vi "CS POLARIS BME DG.configure objects.vi"(8 "error in (no error)":errorcluster, 11 "BME_DG_System in":refnum<class "BME_DG_System.lvclass">) -> (0 "error out":errorcluster, 3 "BME_DG_System out":refnum<class "BME_DG_System.lvclass">)   [LabVIEW 2009, in "CS POLARIS BME DG.lvlib"]
uses:
  CS POLARIS BME DG.lvlib
  LV-BME Interface/ChnlSettings.ctl
  DG Classes/BME_DG_G05P2/SG05P2 Clock and Trigger Settings.ctl
  LV-BME Interface/BME_DG_TriggerSettings.ctl
  LV-BME Interface/ClockSource.ctl
  DG Classes/BME_DG_System/BME_DG_System.lvclass
  ChnlParam.ctl
  DG Classes/BME_DG_Base/BME_DG_Base.lvclass
  DG Classes/BME_DG_Chnl/BME_DG_Chnl.lvclass
  POLARIS BME DG.lvlib
panel:
  in  "Karten Parameter":T1[](array[typedef])=[{"Trigger"={"InputTerminated?"=FALSE, "InternalClockPeriode(µs)"=1000000.0, "TriggerLevel"=1.25, "PresetValue"=0, "DivideBy"=1, "Clock Source"=1, "Gate Divider"=1, "PositiveGate?"=TRUE, "InternalTrigger?"=TRUE, "InternalArm?"=FALSE, "SWTrigger?"=FALSE, "RisingEdge?"=FALSE, "StopOnPreset?"=FALSE, "ResetWhenDone?"=TRUE, "TriggerEnabled?"=TRUE}, "ClockSource "=1, "V2 Trigger Settings"={"Gate Type"=TRUE, "Synchronize Gate"=FALSE, "Force Trigger (µs)"=0.0, "MS Bus"=16}, " prescaller crst oscill."=8, "CardName"="Master"}, {"Trigger"={"InputTerminated?"=TRUE, "InternalClockPeriode(µs)"=0.0, "TriggerLevel"=1.25, "PresetValue"=0, "DivideBy"=1, "Clock Source"=3, "Gate Divider"=1, "PositiveGate?"=TRUE, "InternalTrigger?"=FALSE, "InternalArm?"=FALSE, "SWTrigger?"=FALSE, "RisingEdge?"=FALSE, "StopOnPreset?"=FALSE, "ResetWhenDone?"=FALSE, "TriggerEnabled?"=FALSE}, "ClockSource "=4, "V2 Trigger Settings"={"Gate Type"=TRUE, "Synchronize Gate"=FALSE, "Force Trigger (µs)"=0.0, "MS Bus"=16}, " prescaller crst oscill."=1, "CardName"="S1"}, {"Trigger"={"InputTerminated?"=TRUE, "InternalClockPeriode(µs)"=0.0, "TriggerLevel"=1.25, "PresetValue"=0, "DivideBy"=1, "Clock Source"=3, "Gate Divider"=1, "PositiveGate?"=TRUE, "InternalTrigger?"=FALSE, "InternalArm?"=FALSE, "SWTrigger?"=FALSE, "RisingEdge?"=FALSE, "StopOnPreset?"=FALSE, "ResetWhenDone?"=FALSE, "TriggerEnabled?"=TRUE}, "ClockSource "=1, "V2 Trigger Settings"={"Gate Type"=TRUE, "Synchronize Gate"=FALSE, "Force Trigger (µs)"=0.0, "MS Bus"=16}, " prescaller crst oscill."=1, "CardName"="S2"}] {"V2 Trigger Settings"."MS Bus" format="%04x" items=["Local Primary"=1, "Local Secondary"=2, "Local Force"=4, "Resynchronize"=8, "Master Primary"=16, "Master Secondary"=32, "Master Force"=64, "System Clock"=128, "Delay Clock"=256, "Inhibit Local"=512, "Start Local"=1024, "Start Bus"=2048, "Step Back Local"=4096, "Step Back Bus"=8192, "Enable From E"=65536, "Enable From F"=131072, "Enable From Bus"=262144]; "V2 Trigger Settings"."Force Trigger (µs)" min=0.0 format="%.6f"; "ClockSource" items=["Internal Oscillator"=1, "External Trigger"=2, "Trigger & Oscillator"=3, "MasterSlave Bus"=4]; "Trigger"."Gate Divider" min=1 max=1000000; "Trigger"."Clock Source" items=["Internal Oscillator"=1, "External Trigger"=2, "Trigger & Oscillator"=3]; "Trigger"."InternalClockPeriode(µs)" format="%#_11g"}
  in  "ChnParam2write":T4={" Delay (µs)"=0.0, "On? (false)"=TRUE, "PositiveVoltage?"=TRUE, "50OhmTerminated? "=TRUE, "25OhmOutput?"=FALSE} {"Delay (µs)" min=0.0 max=100000000.0 format="%.5f"}
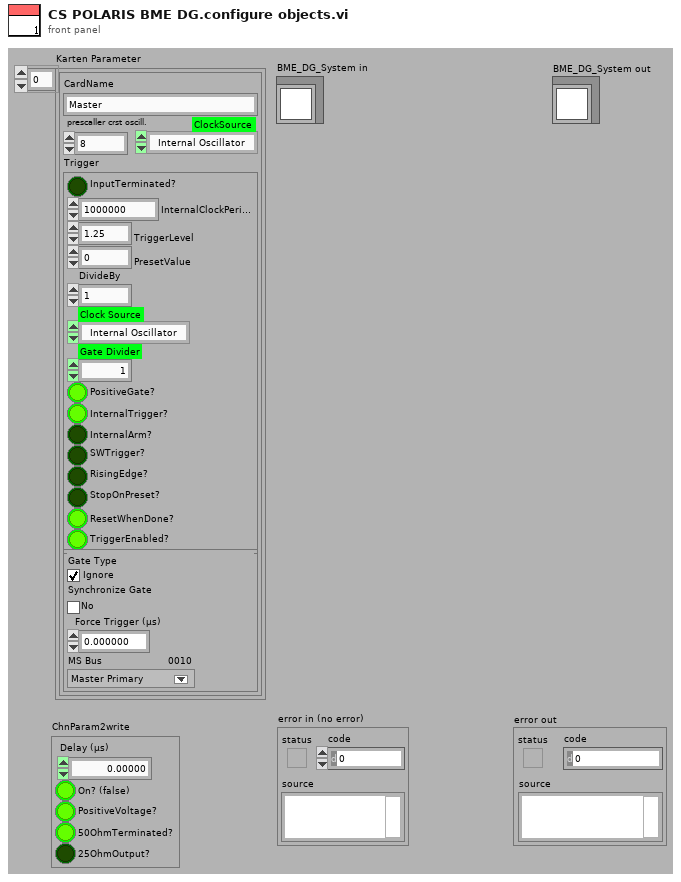
[diagram p1: front panel]
types:
  T1 = typedef "SG05P2 Clock and Trigger Settings.ctl" = cluster{"Trigger":T2, "ClockSource ":T3, "V2 Trigger Settings":cluster{"Gate Type":bool, "Synchronize Gate":bool, "Force Trigger (µs)":dbl, "MS Bus":u32}, " prescaller crst oscill.":u32, "CardName":string}
  T2 = typedef "POLARIS BME DG.lvlib/BME_DG_TriggerSettings.ctl" = cluster{"InputTerminated?":bool, "InternalClockPeriode(µs)":dbl, "TriggerLevel":dbl, "PresetValue":i32, "DivideBy":i32, "Clock Source":u32, "Gate Divider":i32, "PositiveGate?":bool, "InternalTrigger?":bool, "InternalArm?":bool, "SWTrigger?":bool, "RisingEdge?":bool, "StopOnPreset?":bool, "ResetWhenDone?":bool, "TriggerEnabled?":bool}
  T3 = typedef "POLARIS BME DG.lvlib/ClockSource.ctl" = i32
  T4 = typedef "POLARIS BME DG.lvlib/ChnlSettings.ctl" = cluster{" Delay (µs)":dbl, "On? (false)":bool, "PositiveVoltage?":bool, "50OhmTerminated? ":bool, "25OhmOutput?":bool}
  T5 = typedef "ChnlParam.ctl" = cluster{"ChnlName":string, "DelayFormula":string, "OutputModulo":i32}
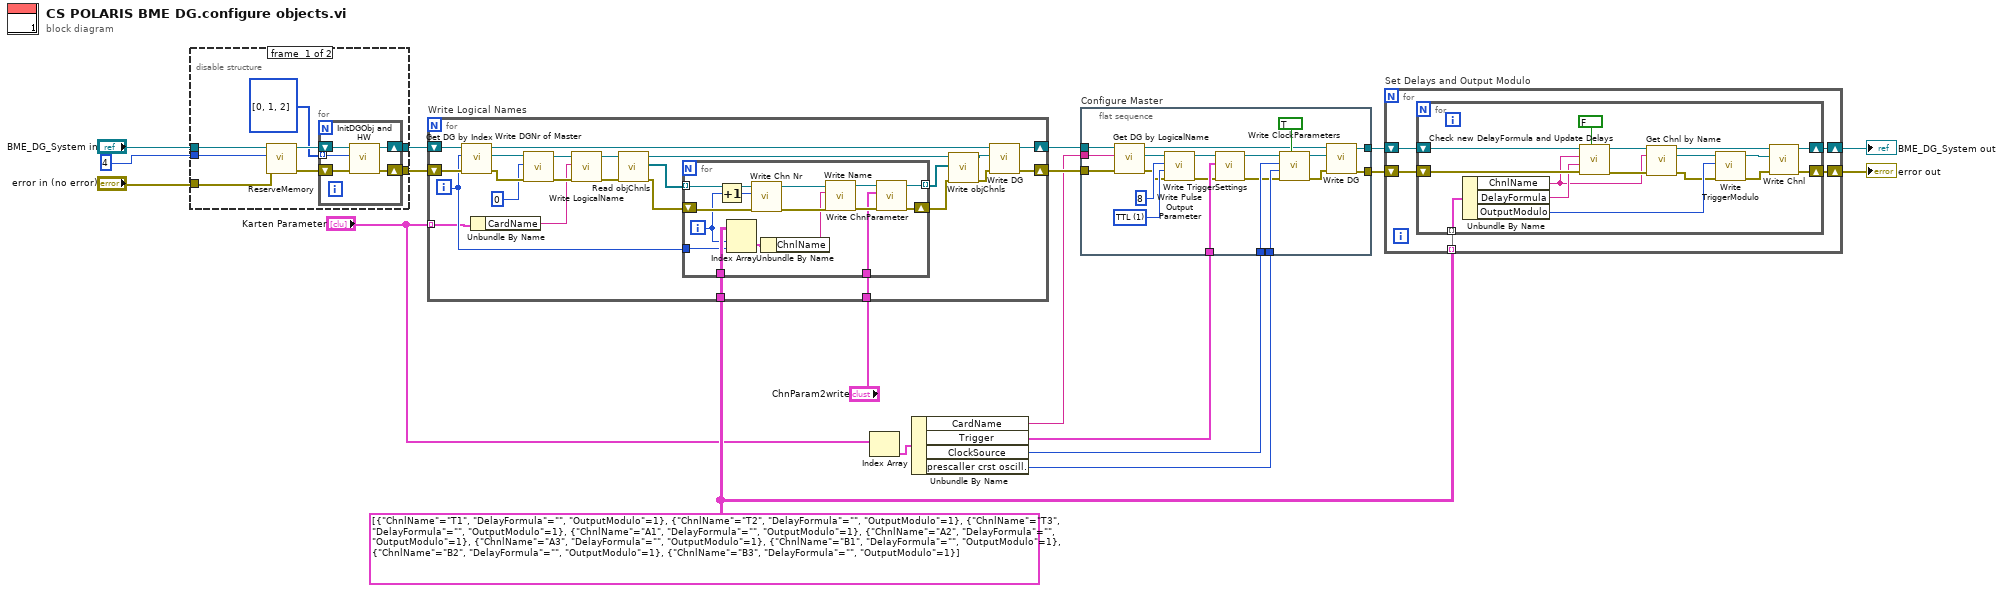
[diagram p0: block diagram]
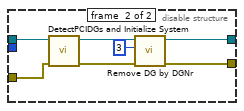
[diagram p2: hidden frame]
diagram:
  w18 = T5[][] [[{"ChnlName"="T1", "DelayFormula"="", "OutputModulo"=1}, {"ChnlName"="T2", "DelayFormula"="", "OutputModulo"=1}, {"ChnlName"="T3", "DelayFormula"="", "OutputModulo"=1}], [{"ChnlName"="A1", "DelayFormula"="", "OutputModulo"=1}, {"ChnlName"="A2", "DelayFormula"="", "OutputModulo"=1}, {"ChnlName"="A3", "DelayFormula"="", "OutputModulo"=1}], [{"ChnlName"="B1", "DelayFormula"="", "OutputModulo"=1}, {"ChnlName"="B2", "DelayFormula"="", "OutputModulo"=1}, {"ChnlName"="B3", "DelayFormula"="", "OutputModulo"=1}]] ("ChnlParam 2")
  n1 = disable-structure shown="Enabled" {
    disable-tunnel: 4 ("#DGs") -> [w25 _]
    disable-tunnel: [w24 w35] -> w6
    disable-tunnel: [w23 w34] -> w5
    disable-tunnel: "BME_DG_System in" -> [w21 w39]
    disable-tunnel: "error in (no error)" -> [w20 w38]
    frame #0 {
      n2 = call "ReserveMemory.vi"("error in (no error)"=w20, "#DGs"=w25, "BME_DG_System in"=w21) -> ("error out"=w26:errorcluster, "BME_DG_System out"=w27:refnum<class "BME_DG_System.lvclass">)  [unwired: 7 in]
      n3 = for {
        tunnel: i32[] [0, 1, 2] -> [w28] mode=indexing
        shift-right: [w30] -> w24
        shift-left: w27 -> [w32]
        shift-right: [w29] -> w23
        shift-left: w26 -> [w31]
        n4 = call "InitDGObj and HW.vi"("error out"=w31, "DGNr"=w28, "BME_DG_System in"=w32) -> ("error IO"=w29:errorcluster, "BME_DG_System Out"=w30:refnum<class "BME_DG_System.lvclass">)  [unwired: 3 in]
      }
    }
    frame #1 {
      n5 = call "DetectPCIDGs and Initialize System.vi"("error in (no error)"=w38, "BME_DG_System in"=w39) -> ("error out"=w36:errorcluster, "BME_DG_System out"=w37:refnum<class "BME_DG_System.lvclass">)  [unwired: 7 in, 1 out]
      n6 = call "Remove DG by DGNr.vi"("error in (no error)"=w36, "DG Nr."=3, "BME_DG_System in"=w37) -> ("error out"=w34:errorcluster, "BME_DG_System out"=w35:refnum<class "BME_DG_System.lvclass">)  [unwired: 5 in, 2 out]
    }
  }
  n7 = for "Write Logical Names" {
    shift-right: [w60] -> w17
    shift-left: w6 -> [w63]
    shift-right: [w59] -> w14
    shift-left: w5 -> [w62]
    tunnel: "ChnParam2write" -> [w56]
    tunnel: w18 -> [w52]
    tunnel: "Karten Parameter" -> [w44] mode=indexing
    i -> [w45]
    n8 = call "Get DG by Index.vi"("error in (no error)"=w62, "index"=w45, "BME_DG_System in"=w63) -> ("error out"=w46:errorcluster, "BME_DG_Base.lvclass"=w49:refnum<class "BME_DG_Base.lvclass">, "BME_DG_System out"=w61:refnum<class "BME_DG_System.lvclass">)  [unwired: 6 in]
    n9 = Unbundle By Name(w44) -> ("CardName"=w43:string)
    n10 = call-dynamic "Write DGNr of Master.vi"("error in (no error)"=w46, "DGNr of Master"=0, "BME_DG_Base in"=w49) -> ("error out"=w47:errorcluster, "BME_DG_Base out"=w48:refnum<class "BME_DG_Base.lvclass">)  [unwired: 7 in]
    n11 = call "Write LogicalName.vi"("error in (no error)"=w47, "LogicalName"=w43, "BME_DG_Base in"=w48) -> ("error out"=w50:errorcluster, "BME_DG_Base out"=w51:refnum<class "BME_DG_Base.lvclass">)  [unwired: 7 in]
    n12 = call-dynamic "Read objChnls.vi"("error in (no error)"=w50, "BME_DG_Base in"=w51) -> ("error out"=w57:errorcluster, "objChnls"=w58:refnum<class "BME_DG_Chnl.lvclass">[], "BME_DG_Base out"=w54:refnum<class "BME_DG_Base.lvclass">)  [unwired: 6 in, 1 out]
    n13 = for {
      tunnel: w58 -> [w75] mode=indexing
      shift-right: [w67] -> w53
      shift-left: w57 -> [w73]
      tunnel: w56 -> [w76]
      tunnel: [w68] -> w55 mode=indexing
      tunnel: w52 -> [w70]
      tunnel: w45 -> [w65]
      i -> [w66]
      n14 = Increment(x=w66) -> (x+1=w71:i32)
      n15 = Index Array(array=w70, index (row)=w66, index (col)=w65) -> (element=w69:T5)
      n16 = call-dynamic "Write Chn Nr.vi"("error in (no error)"=w73, "Chn Nr"=w71, "BME_DG_Chnl in"=w75) -> ("error out"=w72:errorcluster, "BME_DG_Chnl out"=w74:refnum<class "BME_DG_Chnl.lvclass">)  [unwired: 7 in]
      n17 = Unbundle By Name(w69) -> ("ChnlName"=w64:string)
      n18 = call-dynamic "Write Name.vi"("error in (no error)"=w72, "Name"=w64, "BME_DG_Chnl in"=w74) -> ("error out"=w77:errorcluster, "BME_DG_Chnl out"=w78:refnum<class "BME_DG_Chnl.lvclass">)  [unwired: 7 in]
      n19 = call-dynamic "Write ChnParameter.vi"("error in (no error)"=w77, "ChnParemater"=w76, "BME_DG_Chnl in"=w78) -> ("error out"=w67:errorcluster, "BME_DG_Chnl out"=w68:refnum<class "BME_DG_Chnl.lvclass">)  [unwired: 7 in]
    }
    n20 = call-dynamic "Write objChnls.vi"("error in (no error)"=w53, "objChnls"=w55, "BME_DG_Base in"=w54) -> ("error out"=w42:errorcluster, "BME_DG_Base out"=w41:refnum<class "BME_DG_Base.lvclass">)  [unwired: 7 in]
    n21 = call "Write DG.vi"("error in (no error)"=w42, "BME_DG_Base"=w41, "BME_DG_System in"=w61) -> ("error out"=w59:errorcluster, "BME_DG_System out"=w60:refnum<class "BME_DG_System.lvclass">)  [unwired: 7 in]
  }
  n22 = Index Array(array="Karten Parameter") -> (element=w12:T1)  [unwired: 1 in]
  n23 = Unbundle By Name(w12) -> ("CardName"=w11:string, "Trigger"=w10:T2, "ClockSource"=w8:T3, "prescaller crst oscill."=w9:u32)
  n24 = flat-sequence "Configure Master" {
    tunnel: w17 -> [w95]
    tunnel: [w94] -> w16
    tunnel: [w93] -> w15
    tunnel: w14 -> [w92]
    tunnel: w11 -> [w91]
    tunnel: w10 -> [w86]
    tunnel: w8 -> [w85]
    tunnel: w9 -> [w84]
    frame #0 {
      w97 = u32 1 items=["TTL"=1, "NIM"=2, "ECL"=3] ("Pulse Output Level")
      n25 = call "Get DG by LogicalName.vi"("error in (no error)"=w92, "LogicalName"=w91, "BME_DG_System in"=w95) -> ("error out"=w88:errorcluster, "BME_DG_Base.lvclass"=w90:refnum<class "BME_DG_Base.lvclass">, "BME_DG_System out"=w83:refnum<class "BME_DG_System.lvclass">)  [unwired: 5 in, 1 out]
      n26 = call-dynamic "Write Pulse Output Parameter.vi"("error in (no error)"=w88, "Pulse Output Level"=w97, "Pulse Width"=u32 8, "BME_DG_Base in"=w90) -> ("error out"=w81:errorcluster, "BME_DG_Base out"=w82:refnum<class "BME_DG_Base.lvclass">)  [unwired: 6 in]
      n27 = call-dynamic "Write TriggerSettings.vi"("error in (no error)"=w81, "Trigger Settings"=w86, "BME_DG_Base in"=w82) -> ("error out"=w80:errorcluster, "BME_DG_Base out"=w79:refnum<class "BME_DG_Base.lvclass">)  [unwired: 7 in]
      n28 = call-dynamic "Write ClockParameters.vi"("ClockEnable"=TRUE, "error in (no error)"=w80, "PrescalerCrystalOscilator"=w84, "ClockSource"=w85, "BME_DG_Base in"=w79) -> ("error out"=w87:errorcluster, "BME_DG_Base out"=w89:refnum<class "BME_DG_Base.lvclass">)  [unwired: 5 in]
      n29 = call "Write DG.vi"("error in (no error)"=w87, "BME_DG_Base"=w89, "BME_DG_System in"=w83) -> ("error out"=w93:errorcluster, "BME_DG_System out"=w94:refnum<class "BME_DG_System.lvclass">)  [unwired: 7 in]
    }
  }
  n30 = for "Set Delays and Output Modulo" {
    shift-right: [w102] -> w2
    shift-left: w16 -> [w103]
    shift-right: [w100] -> w1
    shift-left: w15 -> [w101]
    tunnel: w18 -> [w99] mode=indexing
    n31 = for {
      shift-right: [w110] -> w102
      shift-left: w103 -> [w119]
      shift-right: [w109] -> w100
      shift-left: w101 -> [w118]
      tunnel: w99 -> [w116] mode=indexing
      n32 = Unbundle By Name(w116) -> ("ChnlName"=w112:string, "DelayFormula"=w115:string, "OutputModulo"=w111:i32)
      n33 = call "Check new DelayFormula and Update Delays.vi"("Update HW"=FALSE, "error in (no error)"=w118, "Delay Formula"=w115, "ChnlName"=w112, "BME_DG_System in"=w119) -> ("error out"=w113:errorcluster, "BME_DG_System out"=w114:refnum<class "BME_DG_System.lvclass">)  [unwired: 4 in, 1 out]
      n34 = call "Get Chnl by Name.vi"("BME_DG_System in"=w114, "Chnl Name"=w112, "error in (no error)"=w113) -> ("BME_DG_System out"=w108:refnum<class "BME_DG_System.lvclass">, "BME_DG_Chnl"=w104:refnum<class "BME_DG_Chnl.lvclass">, "error out"=w105:errorcluster)  [unwired: 7 in, 3 out]
      n35 = call-dynamic "Write TriggerModulo.vi"("error in (no error)"=w105, "TriggerModulo"=w111, "BME_DG_G05_Chnl in"=w104) -> ("error out"=w107:errorcluster, "BME_DG_G05_Chnl out"=w106:refnum<class "BME_DG_Chnl.lvclass">)  [unwired: 7 in]
      n36 = call "Write Chnl.vi"("error in (no error)"=w107, "BME_DG_Chnl.lvclass"=w106, "BME_DG_System in"=w108) -> ("error out"=w109:errorcluster, "BME_DG_System out"=w110:refnum<class "BME_DG_System.lvclass">)  [unwired: 7 in]
    }
  }
  "BME_DG_System out" <- w2
  "error out" <- w1
